vi "exercici contar galetes-2.vi"() -> ()   [LabVIEW 2017]
panel:
  out "Step Status":bool
  out "Results":cluster{i32, i32, i32[]}[](graph)
  in  "Lower Limit":i32
  in  "Upper Limit":i32
  in  "Number of Supremes":i32
  in  "Number of Cups":i32
  in  "Number of Nougats":i32
  in  "Number of Truffles":i32
  in  "Numbers of Caramels":i32
  # "Truffles"
  # "Cups"
  # "Supremes"
  # "Caramels"
  # "Nougats"
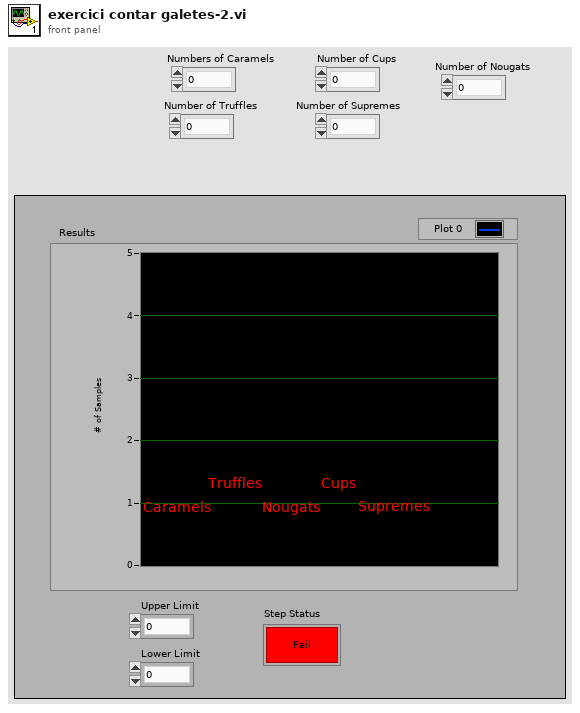
[diagram p1: front panel]
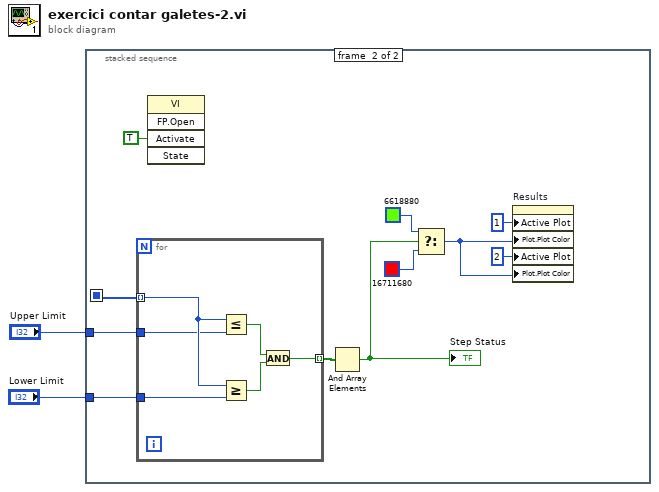
[diagram p0: block diagram]
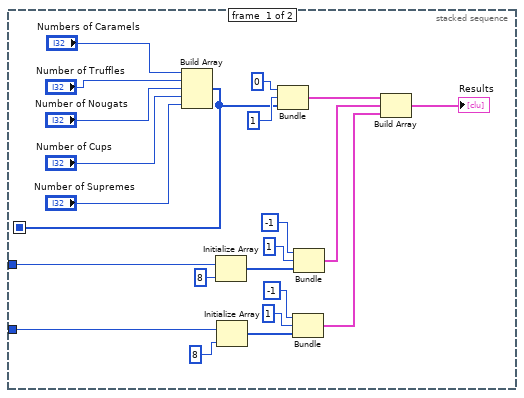
[diagram p2: hidden frame]
diagram:
  n1 = stacked-sequence {
    seq-local: [w17 _] -> [_ w35]
    tunnel: "Lower Limit" -> [w15 w33]
    tunnel: "Upper Limit" -> [w14 w34]
    frame #0 {
      n2 = Build Array "Build Array"("Numbers of Caramels", "Number of Truffles", "Number of Nougats", "Number of Cups", "Number of Supremes") -> (w17:i32[])
      n3 = Initialize Array "Initialize Array"(w14, 8 ("dimension size")) -> (w11:i32[])
      n4 = Initialize Array(w15, 8 ("dimension size")) -> (w10:i32[])
      n5 = Bundle(0, 1, w17) -> (w16:cluster{i32, i32, i32[]})  [unwired: 1 in]
      n6 = Bundle(-1, 1, w10) -> (w4:cluster{i32, i32, i32[]})  [unwired: 1 in]
      n7 = Bundle(-1, 1, w11) -> (w5:cluster{i32, i32, i32[]})  [unwired: 1 in]
      n8 = Build Array(w16, w5, w4) -> (→"Results":cluster{i32, i32, i32[]}[])
    }
    frame #1 {
      n9 = for {
        tunnel: w35 -> [w41] mode=indexing
        tunnel: w34 -> [w40]
        tunnel: w33 -> [w39]
        tunnel: [w36] -> w32 mode=indexing
        n10 = Less Or Equal?(x=w41, y=w40) -> (x <= y?=w38:bool)
        n11 = Greater Or Equal?(x=w41, y=w39) -> (x >= y?=w37:bool)
        n12 = And(x=w38, y=w37) -> (x .and. y?=w36:bool)
      }
      n13 = invoke class="VI" method="FP.Open"("Activate"=TRUE ("Activate?")) -> ()  [unwired: 4 in, 5 out]
      n14 = And Array Elements(Boolean array=w32) -> (logical AND=w26:bool)
      "Step Status" <- w26
      n15 = Select(t=u32 6618880 ("Plot.Plot Color"), s=w26, f=u32 16711680 ("Plot.Plot Color")) -> (s? t:f=w27:u32)
      n16 = property on="Results" class="WFGraph (strict)"("Active Plot"=u32 1, "Plot.Plot Color"=w27, "Active Plot"=u32 2, "Plot.Plot Color"=w27) -> ()  [unwired: 2 in, 2 out]
    }
  }
